vi "SendImage.vi"(1 "ImageClusterRef":T1, 2 "port(3613)":u32=3613, 3 "IP":string, 4 "连接ID":refnum<k16>) -> (0 "长度":i32)   [LabVIEW 2012]
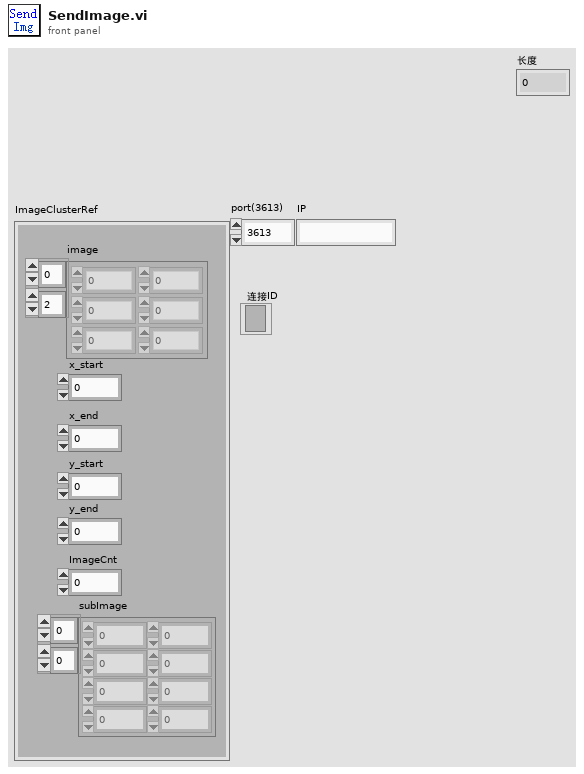
[diagram p1: front panel]
types:
  T1 = cluster{"image":i16[][], "x_start":u32, "x_end":u32, "y_start":u32, "y_end":u32, "ImageCnt":u32, "subImage":u16[][]}
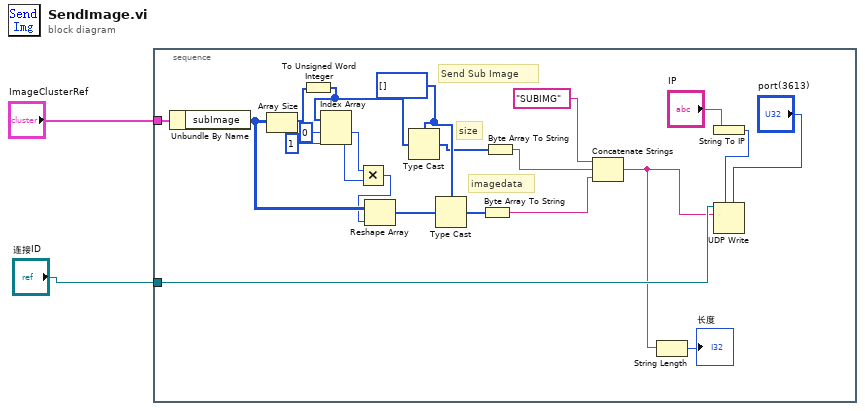
[diagram p0: block diagram]
diagram:
  n1 = stacked-sequence {
    tunnel: "ImageClusterRef" -> [w24]
    tunnel: "连接ID" -> [w5]
    frame #0 {
      w14 = u8[] []
      # "imagedata"
      # "size"
      # "Send Sub Image"
      n2 = Unbundle By Name(w24) -> ("subImage"=w19:u16[][])
      n3 = Array Size(array=w19) -> (size(s)=w21:i32[])
      n4 = To Unsigned Word Integer(number=w21) -> (unsigned 16bit integer=w20:u16[])
      n5 = Index Array(array=w20, index #1=0 ("索引"), index #2=1 ("索引")) -> (element #1=w18:u16, element #2=w17:u16)
      n6 = Multiply(x=w18, y=w17) -> (x*y=w16:u16)
      n7 = Reshape Array(w19, w16) -> (w15:u16[])
      n8 = Type Cast(type=w14, x=w20) -> (*(type *) &x=w12:u8[])
      n9 = Type Cast(type=w14, x=w15) -> (*(type *) &x=w13:u8[])
      n10 = Byte Array To String(unsigned byte array=w13) -> (string=w9:string)
      n11 = Byte Array To String(unsigned byte array=w12) -> (string=w10:string)
      n12 = Concatenate Strings("SUBIMG", w10, w9) -> (w4:string)
      n13 = String Length(string=w4) -> (length=→"长度":i32)
      n14 = String To IP(1:"IP") -> (0:w7:u32)
      n15 = UDP Write(address=w7, port or service name="port(3613)", connection ID=w5, data in=w4) -> ()  [unwired: 2 in, 2 out]
    }
  }
